vi "Write 1D I32.vi"(7 "count (-1: all)":i64=-1 format="%d elements", 8 "error in (no error)":errorcluster, 9 "offset (0)":u64 format="%d bytes", 10 "buffer in":i32[](array[numeric]), 11 "Pointer in":refnum<class "Pointer.lvclass">) -> (0 "error out":errorcluster, 1 "offset + size":u64 format="%d bytes", 2 "buffer out":i32[](array[numeric]), 3 "Pointer out":refnum<class "Pointer.lvclass">)   [LabVIEW 2027, in "Memory Manager.lvlib" / "Pointer.lvclass"]
doc: "Writes <b>count</b> elements from the provided <b>buffer</b> to the address specified by <b>pointer + offset</b>."
uses:
  Pointer.lvclass
  Write (No Check) 1D I32.vi
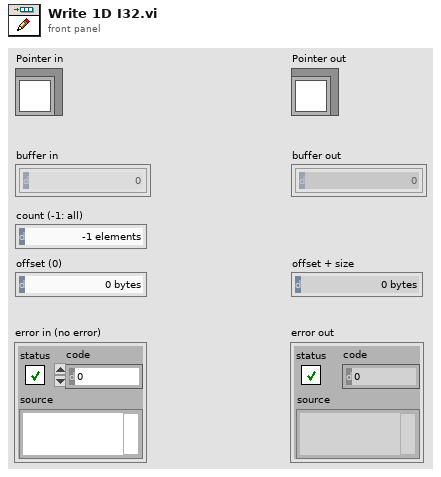
[diagram p1: front panel]
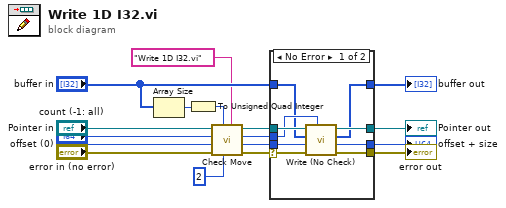
[diagram p0: block diagram]
diagram:
  n1 = Array Size(array="buffer in") -> (size(s)=w17:i32)
  n2 = To Unsigned Quad Integer(1:w17) -> (0:w12:u64)
  n3 = call "Check Move.vi"("source vi name"="Write 1D I32.vi", "count power of 2"=u8 2, "buffer count"=w12, "error in (no error)"="error in (no error)", "offset (0)"="offset (0)", "move count (-1: rest)"="count (-1: all)", "Pointer in"="Pointer in") -> ("error out"=w15:errorcluster, "offset"=w14:u64, "count"=w13:u64, "Pointer out"=w16:refnum<class "Pointer.lvclass">)  [unwired: 1 in]
  n4 = case shown="No Error" w15 {
    selector: w15 -> [w26 w29]
    tunnel: w16 -> [w24 w28]
    tunnel: w14 -> [w25 w30]
    tunnel: "buffer in" -> [w18 w27]
    tunnel: [w23 w29] -> w7
    tunnel: [w22 w28] -> w8
    tunnel: [w21 w30] -> w2
    tunnel: [w20 w27] -> w5
    tunnel: w13 -> [w19 _]
    frame No Error {
      n5 = call-poly "Write (No Check).vi"("count"=w19, "error in (no error)"=w26, "offset (0)"=w25, "buffer in"=w18, "Pointer in"=w24) -> ("error out"=w23:errorcluster, "offset + size"=w21:u64, "buffer out"=w20:i32[], "Pointer out"=w22:refnum<class "Pointer.lvclass">)  [unwired: 3 in]
    }
    frame Error {
    }
  }
  "error out" <- w7
  "Pointer out" <- w8
  "buffer out" <- w5
  "offset + size" <- w2
